vi "polarizador.vi"(8 "Velocidad":dbl, 9 "Angulo":dbl, 10 "SerialNumber":string) -> (0 "error out":errorcluster, 3 "Angulo salida":i32)   [LabVIEW 2016]
uses:
  C:/Users/Posgrado/Desktop/Camara y mapeo/rot/Thorlabs.MotionControl.IntegratedStepperMotorsCLI.dll
  rot/Thorlabs.MotionControl.IntegratedStepperMotorsCLI.dll
  C:/Users/Posgrado/Desktop/Camara y mapeo/rot/Thorlabs.MotionControl.Controls.dll
  rot/Thorlabs.MotionControl.Controls.dll
panel:
  in  "CageRotatorControl":refnum<k24>(container)
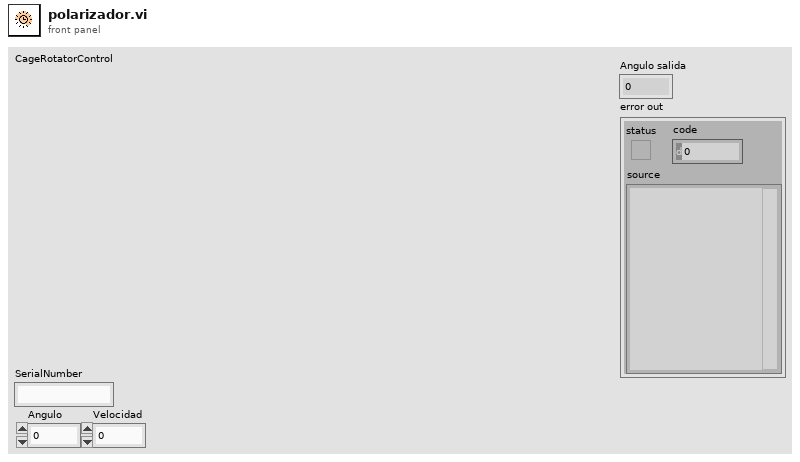
[diagram p1: front panel]
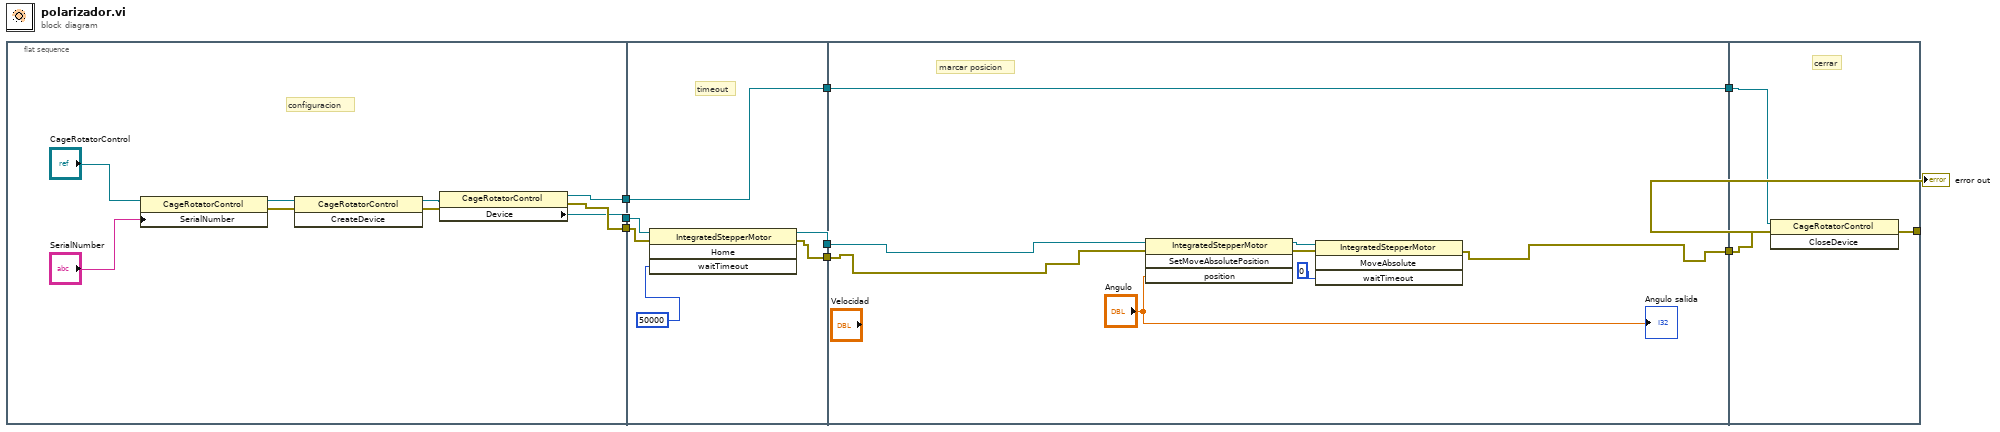
[diagram p0: block diagram]
diagram:
  n1 = flat-sequence {
    tunnel: [w13] -> w9
    tunnel: [w11] -> w8
    tunnel: [w12] -> w7
    tunnel: w9 -> [w24]
    tunnel: w8 -> [w21]
    tunnel: w7 -> [w20]
    tunnel: [w24] -> w6
    tunnel: [w23] -> w5
    tunnel: [w22] -> w1
    tunnel: w6 -> [w32]
    tunnel: w5 -> [w28]
    tunnel: [w32] -> w4
    tunnel: [w26] -> w3
    tunnel: w1 -> [w27]
    tunnel: w4 -> [w35]
    tunnel: w3 -> [w34]
    tunnel: [w33] -> w2
    frame #0 {
      # "configuracion"
      n2 = property class="CageRotatorControl"(reference="CageRotatorControl", "SerialNumber"="SerialNumber") -> (reference out=w16:refnum<k24>, error out=w15:errorcluster)  [unwired: 1 in]
      n3 = invoke class="CageRotatorControl" method="CreateDevice"(reference=w16, error in=w15) -> (reference out=w14:refnum<k24>, error out=w10:errorcluster)  [unwired: 1 in, 1 out]
      n4 = property class="CageRotatorControl"(reference=w14, error in=w10) -> (reference out=w13:refnum<k24>, error out=w12:errorcluster, "Device"=w11:refnum<k24>)
    }
    frame #1 {
      # "timeout"
      n5 = invoke class="IntegratedStepperMotor" method="Home"(reference=w21, error in=w20, "waitTimeout"=50000) -> (reference out=w23:refnum<k24>, error out=w22:errorcluster)  [unwired: 1 in, 2 out]
    }
    frame #2 {
      # "marcar posicion"
      n6 = invoke class="IntegratedStepperMotor" method="SetMoveAbsolutePosition"(reference=w28, error in=w27, "position"="Angulo") -> (reference out=w31:refnum<k24>, error out=w30:errorcluster)  [unwired: 1 in, 2 out]
      n7 = invoke class="IntegratedStepperMotor" method="MoveAbsolute"(reference=w31, error in=w30, "waitTimeout"=0) -> (error out=w26:errorcluster)  [unwired: 1 in, 3 out]
      "Angulo salida" <- "Angulo"
    }
    frame #3 {
      # "cerrar"
      n8 = invoke class="CageRotatorControl" method="CloseDevice"(reference=w35, error in=w34) -> (error out=w33:errorcluster)  [unwired: 1 in, 2 out]
    }
  }
  "error out" <- w2
